vi "Audio.Generate DTMF Phone Num Keys.vi"(11 "DTMF Num":i32) -> (3 "tones":T1(array[cluster])=[{"frequency"=1000.0, "amplitude"=1.0, "phase"=0.0}])   [LabVIEW 2018]
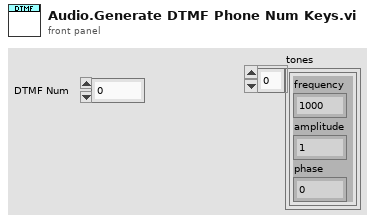
[diagram p1: front panel]
types:
  T1 = cluster{"frequency":dbl, "amplitude":dbl, "phase":dbl}[]
  T2 = cluster{"frequency":dbl, "amplitude":dbl, "phase":dbl}
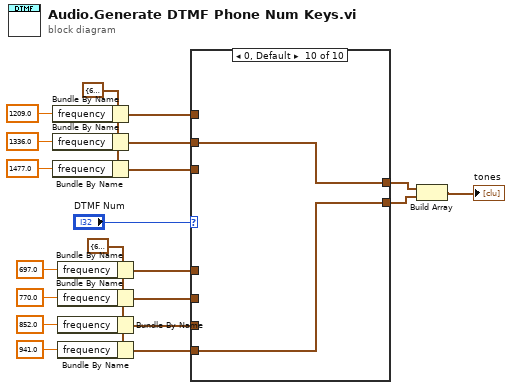
[diagram p0: block diagram]
diagram:
  w15 = T2 {"frequency"=697.0, "amplitude"=1.0, "phase"=0.0} ("tone f, a, p")
  w16 = T2 {"frequency"=697.0, "amplitude"=1.0, "phase"=0.0} ("tone f, a, p")
  n1 = Bundle By Name(cluster=w15, "frequency"=1209.0) -> (w10:T2)
  n2 = Bundle By Name(cluster=w15, "frequency"=1336.0) -> (w9:T2)
  n3 = Bundle By Name(cluster=w15, "frequency"=1477.0) -> (w8:T2)
  n4 = Bundle By Name(cluster=w16, "frequency"=697.0) -> (w7:T2)
  n5 = Bundle By Name(cluster=w16, "frequency"=770.0) -> (w6:T2)
  n6 = Bundle By Name(cluster=w16, "frequency"=852.0) -> (w5:T2)
  n7 = Bundle By Name(cluster=w16, "frequency"=941.0) -> (w4:T2)
  n8 = case shown="0, Default" "DTMF Num" {
    tunnel: w10 -> [w21 _ _ w27 _ _ w33 _ _ _]
    tunnel: w9 -> [_ w23 _ _ w29 _ _ w35 _ w40]
    tunnel: w8 -> [_ _ w25 _ _ w31 _ _ w38 _]
    tunnel: w7 -> [w22 w24 w26 _ _ _ _ _ _ _]
    tunnel: w6 -> [_ _ _ w28 w30 w32 _ _ _ _]
    tunnel: w5 -> [_ _ _ _ _ _ w34 w36 w37 _]
    tunnel: w4 -> [_ _ _ _ _ _ _ _ _ w39]
    tunnel: [w22 w24 w26 w28 w30 w32 w34 w36 w37 w39] -> w2
    tunnel: [w21 w23 w25 w27 w29 w31 w33 w35 w38 w40] -> w1
    frame 1 {
    }
    frame 2 {
    }
    frame 3 {
    }
    frame 4 {
    }
    frame 5 {
    }
    frame 6 {
    }
    frame 7 {
    }
    frame 8 {
    }
    frame 9 {
    }
    frame 0, Default {
    }
  }
  n9 = Build Array(w1, w2) -> (→"tones":T1)
